vi "soil moisture for integrtaed.vi"(6 "stop for soilmoisture":bool, 7 "PwmpinLedMoisture":u8, 8 "Error Out":errorcluster, 9 "Analog Channe for soil moisturel":u8, 10 "Pumppin":u8, 11 "LINX Resource":T1) -> (0 "Error Out 2":errorcluster, 3 "LINX Resource 2":T1, 5 "Waveform Chart moisture":dbl(graph))   [LabVIEW 2020]
uses:
  <vilib>/MakerHub/LINX/Private/Type Defs/LINX Ref.ctl
  <vilib>/MakerHub/LINX/Private/Type Defs/Platform.ctl
  <vilib>/MakerHub/LINX/Private/Type Defs/Interface.ctl
  <vilib>/MakerHub/LINX/Private/Device/Type Defs/LINX Device Config.ctl
  <vilib>/MakerHub/LINX/Private/Device/Type Defs/TCP Config.ctl
  <vilib>/MakerHub/LINX/Private/Device/Type Defs/Channels.ctl
  <vilib>/MakerHub/LINX/Public/Peripherals/Analog/Analog Read 1 Chan.vi
  <vilib>/MakerHub/LINX/Public/Peripherals/PWM/PWM Set Duty Cycle 1 Chan.vi
  <vilib>/MakerHub/LINX/Public/Peripherals/Digital/Digital Write 1 Chan.vi
  <vilib>/MakerHub/LINX/Public/Peripherals/Analog/Analog Read N Chans.vi
  <vilib>/MakerHub/LINX/Public/Peripherals/Digital/Digital Write N Chans.vi
  <vilib>/MakerHub/LINX/Private/Local IO/LinxAnalogRead.vi
  <vilib>/MakerHub/LINX/Public/Utilities/Check Channel.vi
  <vilib>/MakerHub/LINX/Private/Local IO/LinxDigitalWrite.vi
  <vilib>/MakerHub/LINX/Private/Utilties/Generate Error.vi
  <vilib>/MakerHub/LINX/Public/Peripherals/PWM/PWM Set Duty Cycle N Chans.vi
  <vilib>/MakerHub/LINX/LMH-LINX.lvlib
  <vilib>/MakerHub/LINX/Private/Device/Device.lvlib
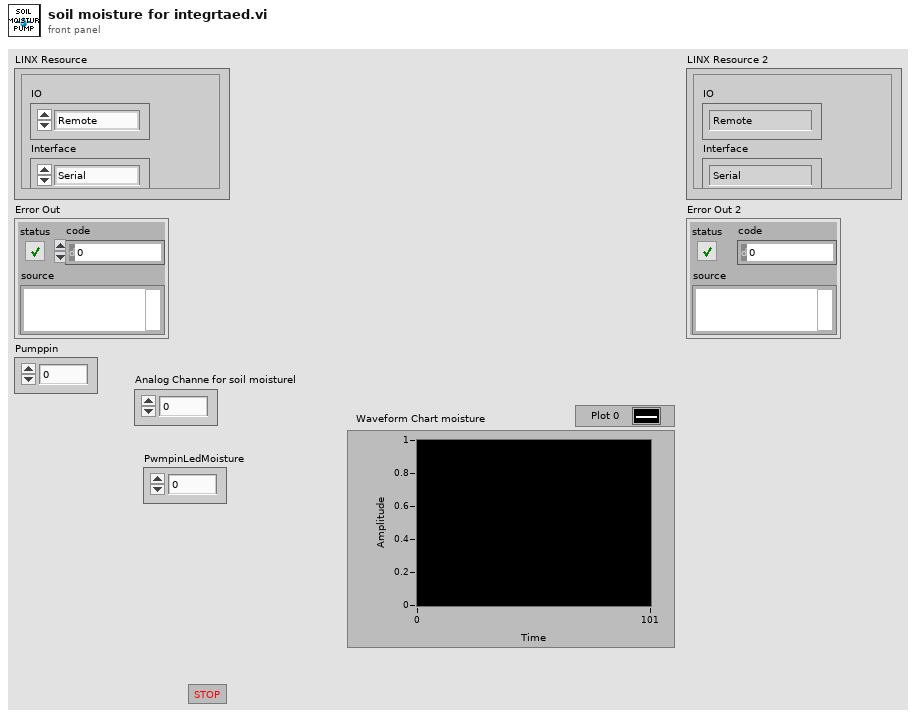
[diagram p1: front panel]
types:
  T1 = typedef "LMH-LINX.lvlib/LINX Ref.ctl" = cluster{"IO":T2, "Interface":T3, "LINX Device Config":T4}
  T2 = typedef "LMH-LINX.lvlib/Platform.ctl" = enum16{"Remote", "Local"}
  T3 = typedef "LMH-LINX.lvlib/Interface.ctl" = enum16{"Serial", "TCP"}
  T4 = typedef "LMH-LINX.lvlib/Device.lvlib/LINX Device Config.ctl" = cluster{"Interface":T3, "COM Port":refnum<visa-resource-name>, "TCP Configuration":T5, "Device Family":u8, "Device ID":u8, "Device Name":string, "TCP Ref":refnum<k5>, "Channels":T6}
  T5 = typedef "LMH-LINX.lvlib/Device.lvlib/TCP Config.ctl" = cluster{"IP Address":string, "Port":u16}
  T6 = typedef "LMH-LINX.lvlib/Channels.ctl" = cluster{"DI":u8[], "DO":u8[], "AI":u8[], "AO":u8[], "PWM":u8[], "QE":u8[], "UART":u8[], "I2C 2":u8[], "SPI":u8[], "CAN":u8[], "Servo":u8[], "AI Ref (V)":dbl, "AI Resolution (Bits)":u8, "AO Ref (V)":dbl, "AO Resolution (Bits)":u8}
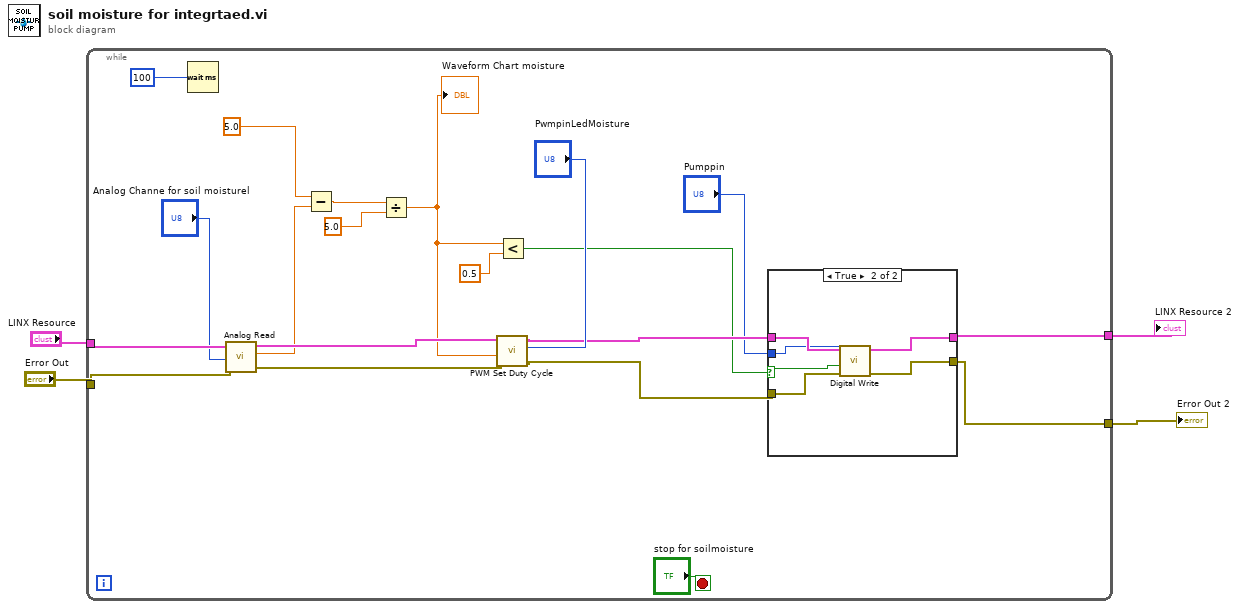
[diagram p0: block diagram]
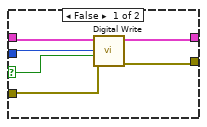
[diagram p2: hidden frame]
diagram:
  n1 = while {
    tunnel: "Error Out" -> [w23]
    tunnel: [w6] -> w4
    tunnel: "LINX Resource" -> [w15]
    tunnel: [w5] -> w3
    stop <- "stop for soilmoisture" stop-if-true
    n2 = Wait (ms)(milliseconds to wait=u32 100 ("millisecond timer value")) -> ()  [unwired: 1 out]
    n3 = call-poly <vilib>:"Analog Read.vi"("Error In"=w23, "Analog Channel"="Analog Channe for soil moisturel", "LINX Resource"=w15) -> ("Error Out"=w20:errorcluster, "Voltage"=w19:dbl, "LINX Resource"=w21:T1)  [unwired: 5 in, 1 out]
    n4 = Subtract(x=5.0, y=w19) -> (x-y=w17:dbl)
    n5 = Divide(x=w17, y=5.0) -> (x/y=w9:dbl)
    "Waveform Chart moisture" <- w9
    n6 = call-poly <vilib>:"PWM Set Duty Cycle.vi"("Error In"=w20, "Duty Cycle (0-1)"=w9, "PWM Channel"="PwmpinLedMoisture", "LINX Resource"=w21) -> ("Error Out"=w11:errorcluster, "LINX Resource"=w12:T1)  [unwired: 6 in]
    n7 = Less?(x=w9, y=0.5) -> (x < y?=w7:bool)
    n8 = case shown="True" w7 {
      selector: w7 -> [w26 w32]
      tunnel: w12 -> [w30 w36]
      tunnel: [w29 w35] -> w6
      tunnel: w11 -> [w27 w34]
      tunnel: [w28 w33] -> w5
      tunnel: "Pumppin" -> [w25 w31]
      frame False {
        n9 = call-poly <vilib>:"Digital Write.vi"("Error In"=w27, "Output Value"=w26, "DO Channel"=w25, "LINX Resource"=w30) -> ("Error Out"=w28:errorcluster, "LINX Resource"=w29:T1)  [unwired: 6 in]
      }
      frame True {
        n10 = call-poly <vilib>:"Digital Write.vi"("Error In"=w34, "Output Value"=w32, "DO Channel"=w31, "LINX Resource"=w36) -> ("Error Out"=w33:errorcluster, "LINX Resource"=w35:T1)  [unwired: 6 in]
      }
    }
  }
  "LINX Resource 2" <- w4
  "Error Out 2" <- w3
